vi "Snake Game.vi"() -> ()   [LabVIEW 2021]
uses:
  Board/Direction.ctl
  Board/Board_Game.lvclass
  Fruit/Fruit.lvclass
  SnakeGame/Snake.lvclass
panel:
  out "Score":u32
  out "Board":u32[][](array[colorbox])
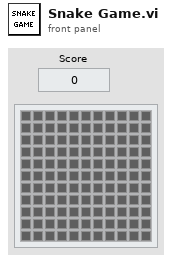
[diagram p1: front panel]
types:
  T1 = typedef "Direction.ctl" = enum16{"Up", "Down", "Left", "Right"}
  T2 = typedef "eventvkey.ctl" = enum16{"ASCII", "Enter", "Return", "Shift", "Ctrl", "Alt", "Cmd", "Opt", "Caps", "NumLock", "Clear", "Break", "Up", "Down", "Left", "Right", "Insert", "Delete", "Home", "End", "PageUp", "PageDown", "Escape", "Help", "Pause", "ScrollLock", "F1", "F2", "F3", "F4", "F5", "F6", "F7", "F8", "F9", "F10", "F11", "F12", "F13", "F14", "F15", "F16", "F17", "F18", "F19", "F20", "F21", "F22", "F23", "F24", "Play", "VolumeUp", "VolumeDown", "Mute", "Two Byte Char"}
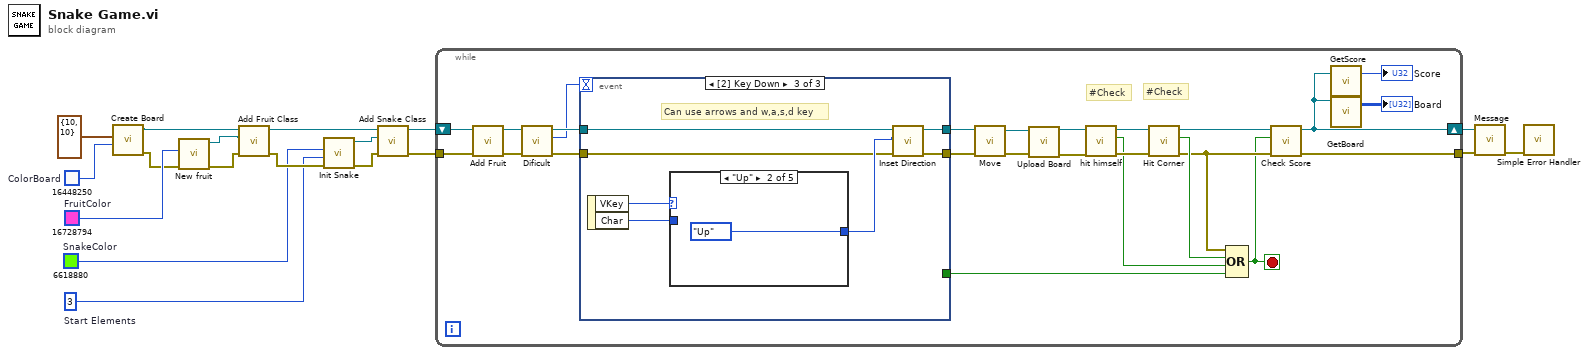
[diagram p0: block diagram]
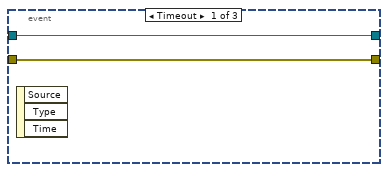
[diagram p2: hidden frame]
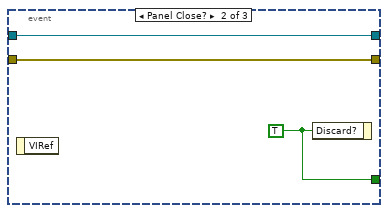
[diagram p3: hidden frame]
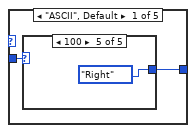
[diagram p4: hidden frame]
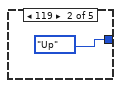
[diagram p6: hidden frame]
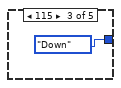
[diagram p7: hidden frame]
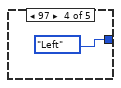
[diagram p8: hidden frame]
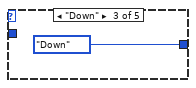
[diagram p9: hidden frame]
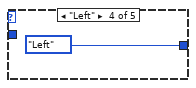
[diagram p10: hidden frame]
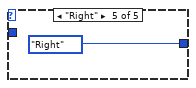
[diagram p11: hidden frame]
diagram:
  w2 = u32 3  # Start Elements
  w3 = u32 6618880  # SnakeColor
  w15 = u32 16448250  # ColorBoard
  w18 = u32 16728794  # FruitColor
  n1 = call "Create Board.vi"("ColorBoard"=w15, "BoardSize"=cluster{"X":i32, "Y":i32} {"X"=10, "Y"=10}) -> ("error out"=w16:errorcluster, "Board_Game out"=w9:refnum<class "Board_Game.lvclass">)  [unwired: 8 in]
  n2 = call "New fruit.vi"("error in (no error)"=w16, "SnakeColor"=w18) -> ("error out"=w10:errorcluster, "Fruit out"=w11:refnum<class "Fruit.lvclass">)  [unwired: 8 in]
  n3 = call-dynamic "Add Fruit Class.vi"("error in (no error)"=w10, "Fruit"=w11, "Board_Game in"=w9) -> ("error out"=w5:errorcluster, "Board_Game out"=w1:refnum<class "Board_Game.lvclass">)  [unwired: 7 in]
  n4 = call "Init Snake.vi"("error in (no error)"=w5, "Start Elements"=w2, "SnakeColor"=w3) -> ("error out"=w4:errorcluster, "Snake out"=w6:refnum<class "Snake.lvclass">)  [unwired: 7 in]
  n5 = call-dynamic "Add Snake Class.vi"("error in (no error)"=w4, "Snake"=w6, "Board_Game in"=w1) -> ("error out"=w7:errorcluster, "Board_Game out"=w8:refnum<class "Board_Game.lvclass">)  [unwired: 7 in]
  n6 = while {
    tunnel: [w31] -> w13
    shift-right: [w28] -> w14
    shift-left: w8 -> [w26]
    tunnel: w7 -> [w40]
    stop <- w29 stop-if-true
    # "#Check"
    # "#Check"
    n7 = call-dynamic "Add Fruit.vi"("error in (no error)"=w40, "Board_Game in"=w26) -> ("error out"=w27:errorcluster, "Board_Game out"=w25:refnum<class "Board_Game.lvclass">)  [unwired: 8 in]
    n8 = call-dynamic "Dificult.vi"("error in (no error)"=w27, "Board_Game in"=w25) -> ("error out"=w35:errorcluster, "Difficult"=w33:i32, "Board_Game out"=w34:refnum<class "Board_Game.lvclass">)  [unwired: 7 in]
    n9 = event shown="[2] Key Down" {
      selector: _ -> [_ _ _]
      dyn-events: _ -> [_ _ _]
      timeout: w33 -> [_ _ _]
      tunnel: [w45 w48 w51] -> w22
      tunnel: w34 -> [w45 w48 w53]
      tunnel: [_ w47 _] -> w43
      tunnel: [w44 w46 w49] -> w20
      tunnel: w35 -> [w44 w46 w50]
      event Timeout {
        n10 = event-data() -> ()  [unwired: 1 in, 3 out]
      }
      event Panel Close? {
        w47 = TRUE ("Discard?")
        n11 = event-data() -> ()  [unwired: 1 in, 1 out]
        n12 = event-data("Discard?"=w47) -> ()  [unwired: 1 in, 1 out]
      }
      event Key Down {
        # "Can use arrows and w,a,s,d key"
        n13 = event-data() -> ("VKey"=w55:T2, "Char"=w54:i16)  [unwired: 1 in]
        n14 = case shown="\"Up\"" w55 {
          tunnel: [w56 Direction."Up" ("Keyboard") Direction."Down" ("Keyboard") Direction."Left" ("Keyboard") Direction."Right" ("Keyboard")] -> w52
          tunnel: w54 -> [w57 _ _ _ _]
          frame "ASCII", Default {
            n15 = case shown="100" w57 {
              tunnel: [_ Direction."Up" ("Keyboard") Direction."Down" ("Keyboard") Direction."Left" ("Keyboard") Direction."Right" ("Keyboard")] -> w56
              frame Default {
              }
              frame 119 {
              }
              frame 115 {
              }
              frame 97 {
              }
              frame 100 {
              }
            }
          }
          frame "Up" {
          }
          frame "Down" {
          }
          frame "Left" {
          }
          frame "Right" {
          }
        }
        n16 = call-dynamic "Inset Direction.vi"("error in (no error)"=w50, "Keyboard"=w52, "Board_Game in"=w53) -> ("error out"=w49:errorcluster, "Board_Game out"=w51:refnum<class "Board_Game.lvclass">)  [unwired: 7 in]
      }
    }
    n17 = call-dynamic "Move.vi"("error in (no error)"=w20, "Board_Game in"=w22) -> ("error out"=w19:errorcluster, "Board_Game out"=w21:refnum<class "Board_Game.lvclass">)  [unwired: 8 in]
    n18 = call-dynamic "Upload Board.vi"("error in (no error)"=w19, "Board_Game in"=w21) -> ("error out"=w24:errorcluster, "Board_Game out"=w23:refnum<class "Board_Game.lvclass">)  [unwired: 8 in]
    n19 = call-dynamic "hit himself.vi"("error in (no error)"=w24, "Board_Game in"=w23) -> ("error out"=w39:errorcluster, "HIT"=w38:bool, "Board_Game out"=w37:refnum<class "Board_Game.lvclass">)  [unwired: 7 in]
    n20 = call-dynamic "Hit Corner.vi"("error in (no error)"=w39, "Board_Game in"=w37) -> ("error out"=w32:errorcluster, "Hit Corner"=w36:bool, "Board_Game out"=w30:refnum<class "Board_Game.lvclass">)  [unwired: 7 in]
    n21 = Compound Arithmetic op=OR(w32, w36, w38, w43) -> (w29:bool)
    n22 = call-dynamic "Check Score.vi"("error in (no error)"=w32, "End"=w29, "Board_Game in"=w30) -> ("error out"=w31:errorcluster, "Board_Game out"=w28:refnum<class "Board_Game.lvclass">)  [unwired: 7 in]
    n23 = call "GetScore.vi"("Board in"=w28) -> ("Score"=→"Score":u32)  [unwired: 1 in]
    n24 = call "GetBoard.vi"("Board in"=w28) -> ("Board"=→"Board":u32[][])  [unwired: 4 in]
  }
  n25 = call "Message.vi"("error in (no error)"=w13, "Board_Game in"=w14) -> ("error out"=w12:errorcluster)  [unwired: 9 in]
  n26 = call <vilib>:"Simple Error Handler.vi"("error in (no error)"=w12) -> ()  [unwired: 4 in, 5 out]
